vi "JOYSTICK1fix.vi"(8 "error in (no error)":errorcluster) -> (0 "error out":errorcluster, 2 "Buttons":bool[](array[boolean]), 3 "Axes":dbl[](array[numeric]), 4 "POVs":i16[](array[numeric]))   [LabVIEW 2017]
panel:
  in  "Scaler":i8=127
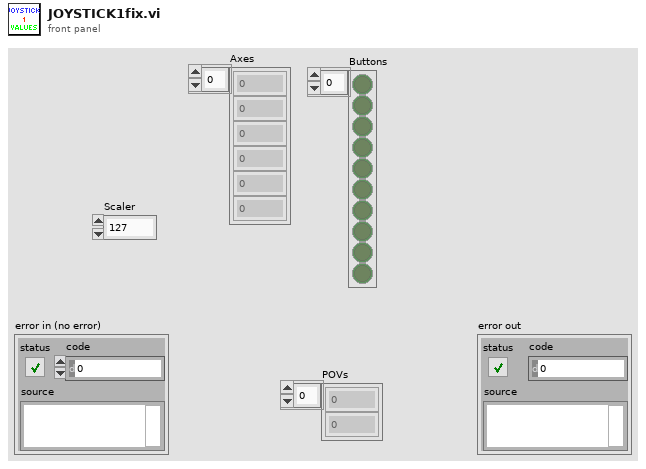
[diagram p1: front panel]
types:
  T1 = enum16{"USB 0", "USB 1", "USB 2", "USB 3", "USB 4", "USB 5"}
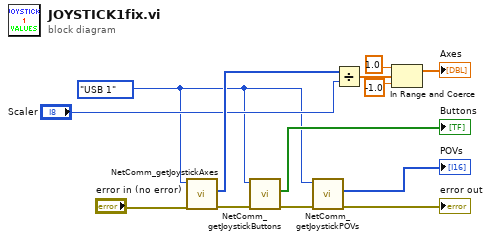
[diagram p0: block diagram]
diagram:
  w1 = T1."USB 1" ("Device")
  n1 = call <vilib>:"NetComm_getJoystickAxes.vi"("error in (no error)"="error in (no error)", "Joystick Number"=w1) -> ("error out"=w10:errorcluster, "Axes"=w8:i16[])  [unwired: 8 in]
  n2 = call <vilib>:"NetComm_getJoystickButtons.vi"("error in (no error)"=w10, "Joystick Number"=w1) -> ("error out"=w9:errorcluster, "Buttons"=→"Buttons":bool[])  [unwired: 8 in]
  n3 = call <vilib>:"NetComm_getJoystickPOVs.vi"("error in (no error)"=w9, "Joystick Number"=w1) -> ("error out"=→"error out":errorcluster, "POVs"=→"POVs":i16[])  [unwired: 8 in]
  n4 = Divide(x=w8, y="Scaler") -> (x/y=w13:dbl[])
  n5 = In Range and Coerce(upper limit=1.0, x=w13, lower limit=-1.0) -> (coerced(x)=→"Axes":dbl[])  [unwired: 1 out]
